vi "helper-windows-control.vi"(6 "Windows Panel":T1 {"EastSideView" scale=0.0..8.0; "WestSideView" scale=0.0..8.0}, 9 "OldVal":variant, 10 "NewVal":variant, 11 "Label.Text":string) -> (0 "error out":errorcluster, 1 "oldVal":i32, 2 "newVal":i32, 3 "canceled?":bool)   [LabVIEW 2024]
uses:
  controls/windows-panel.ctl
panel:
  # "Fully Open"
  # "Fully Close"
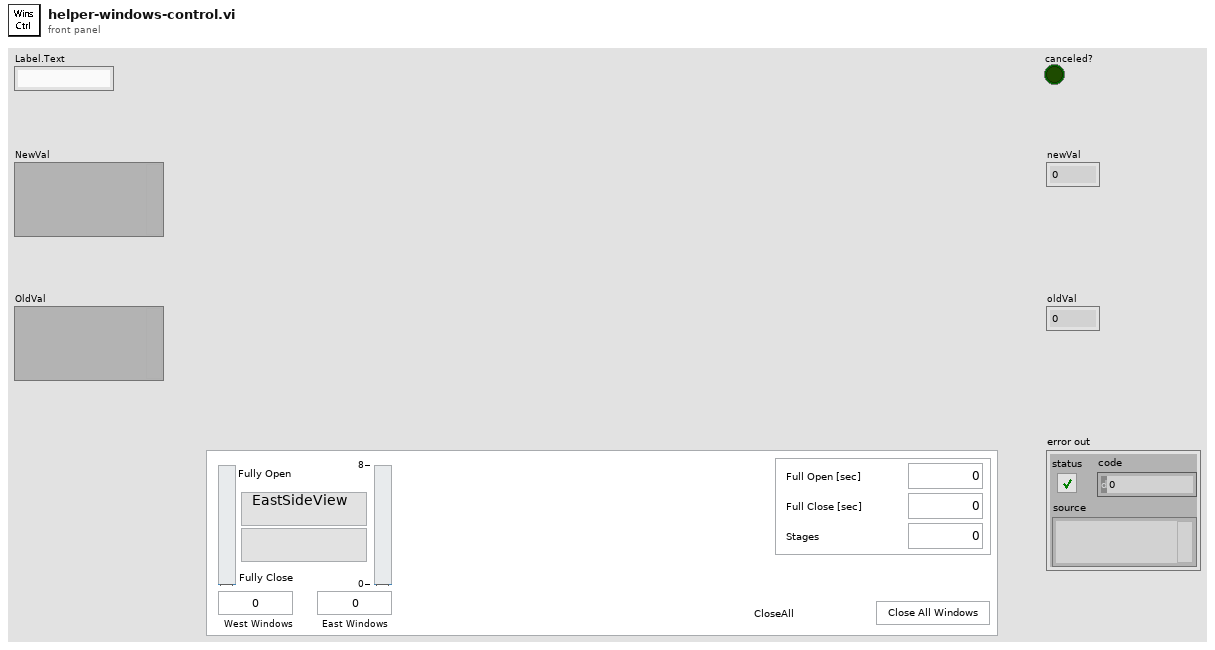
[diagram p1: front panel]
types:
  T1 = typedef "windows-panel.ctl" = cluster{"EastPosition":u16, "WestPosition":u16, "Wind Direction":string, "CloseAll":bool, "WestSideView":u16, "EastSideView":u16, "Wind Speed":string, "confs":cluster{"Full Open [sec]":u16, "Full Close [sec]":u16, "Stages":u16}}
  T2 = enum16{"WINDOWS.EAST.OPEN", "WINDOWS.EAST.CLOSE", "WINDOWS.WEST.OPEN", "WINDOWS.WEST.CLOSE"}
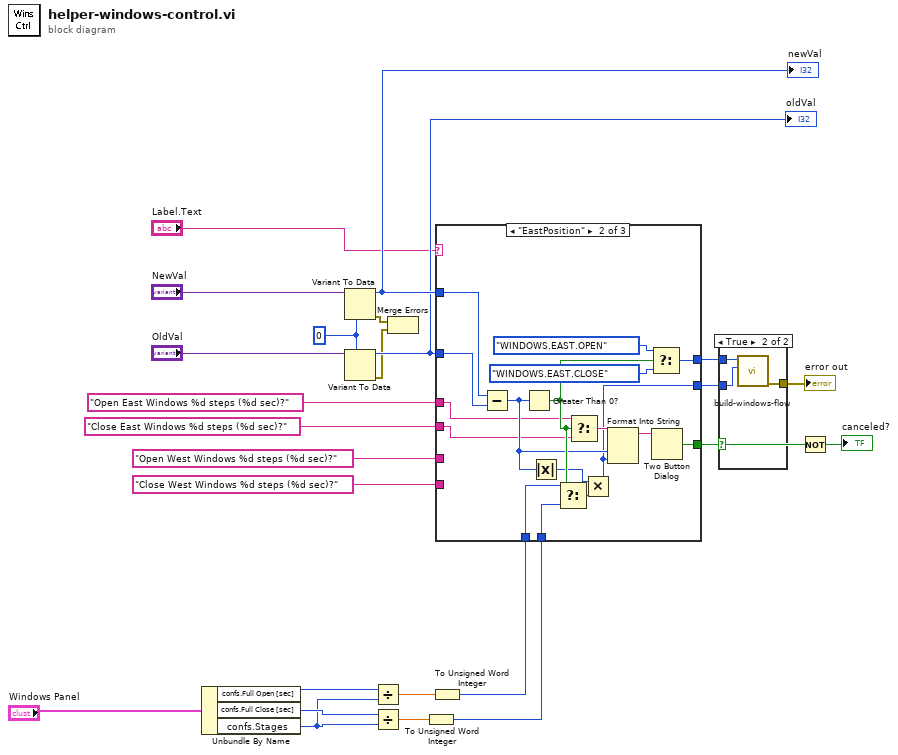
[diagram p0: block diagram]
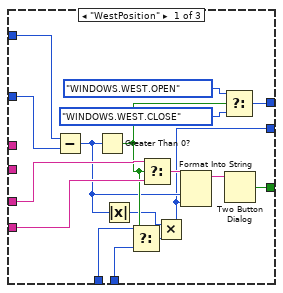
[diagram p3: hidden frame]
diagram:
  w21 = 0
  n1 = Unbundle By Name("Windows Panel") -> ("confs.Full Open [sec]"=w7:u16, "confs.Full Close [sec]"=w6:u16, "confs.Stages"=w5:u16)
  n2 = Variant To Data(type=w21, Variant="NewVal") -> (data=w20:i32, error out=w12:errorcluster)  [unwired: 1 in]
  "newVal" <- w20
  n3 = Variant To Data(type=w21, Variant="OldVal") -> (data=w19:i32, error out=w11:errorcluster)  [unwired: 1 in]
  "oldVal" <- w19
  n4 = Divide(x=w7, y=w5) -> (x/y=w4:dbl)
  n5 = Divide(x=w6, y=w5) -> (x/y=w3:dbl)
  n6 = Merge Errors(w12, w11) -> ()  [unwired: 1 out]
  n7 = To Unsigned Word Integer(number=w3) -> (unsigned 16bit integer=w1:u16)
  n8 = To Unsigned Word Integer(number=w4) -> (unsigned 16bit integer=w2:u16)
  n9 = case shown="\"EastPosition\"" "Label.Text" {
    tunnel: [w38 w55 _] -> w25
    tunnel: [w37 w54 _] -> w24
    tunnel: [w26 w43 _] -> w23
    tunnel: w20 -> [w36 w53 _]
    tunnel: w19 -> [w35 w52 _]
    tunnel: "Open East Windows %d steps (%d sec)?" ("message") -> [_ w45 _]
    tunnel: "Close East Windows %d steps (%d sec)?" ("message") -> [_ w44 _]
    tunnel: "Open West Windows %d steps (%d sec)?" ("message") -> [w34 _ _]
    tunnel: "Close West Windows %d steps (%d sec)?" ("message") -> [w33 _ _]
    tunnel: w2 -> [w31 w50 _]
    tunnel: w1 -> [w30 w49 _]
    frame "WestPosition" {
      n10 = Subtract(x=w36, y=w35) -> (x-y=w28:i32)
      n11 = Greater Than 0?(x=w28) -> (x > 0?=w32:bool)
      n12 = Absolute Value(x=w28) -> (abs(x)=w27:i32)
      n13 = Select(t=w31, s=w32, f=w30) -> (s? t:f=w29:u16)
      n14 = Select(t=w34, s=w32, f=w33) -> (s? t:f=w40:string)
      n15 = Multiply(x=w27, y=w29) -> (x*y=w26:i32)
      n16 = Format Into String(format string=w40, w28, w26) -> (resulting string=w39:string)  [unwired: 2 in, 1 out]
      n17 = Select(t=T2."WINDOWS.WEST.OPEN" ("Operation"), s=w32, f=T2."WINDOWS.WEST.CLOSE" ("Operation")) -> (s? t:f=w37:T2)
      n18 = Two Button Dialog(message=w39) -> (T button?=w38:bool)  [unwired: 2 in]
    }
    frame "EastPosition" {
      n19 = Subtract(x=w53, y=w52) -> (x-y=w47:i32)
      n20 = Greater Than 0?(x=w47) -> (x > 0?=w51:bool)
      n21 = Absolute Value(x=w47) -> (abs(x)=w46:i32)
      n22 = Select(t=w50, s=w51, f=w49) -> (s? t:f=w48:u16)
      n23 = Select(t=w45, s=w51, f=w44) -> (s? t:f=w57:string)
      n24 = Multiply(x=w46, y=w48) -> (x*y=w43:i32)
      n25 = Format Into String(format string=w57, w47, w43) -> (resulting string=w56:string)  [unwired: 2 in, 1 out]
      n26 = Select(t=T2."WINDOWS.EAST.OPEN" ("Operation"), s=w51, f=T2."WINDOWS.EAST.CLOSE" ("Operation")) -> (s? t:f=w54:T2)
      n27 = Two Button Dialog(message=w56) -> (T button?=w55:bool)  [unwired: 2 in]
    }
    frame Default {
    }
  }
  n28 = case shown="True" w25 {
    tunnel: [_ w62] -> w22
    tunnel: w24 -> [_ w61]
    tunnel: w23 -> [_ w60]
    frame False {
    }
    frame True {
      n29 = call "build-windows-flow.vi"("Delay [s]"=w60, "Operation"=w61) -> ("error out"=w62:errorcluster)  [unwired: 8 in, 1 out]
    }
  }
  "error out" <- w22
  n30 = Not(x=w25) -> (.not. x?=→"canceled?":bool)
